vi "Server send.vi"() -> ()   [LabVIEW 2016, in "TCP文件传输系统.lvlib"]
uses:
  <vilib>/Utility/miscctls.llb/LVPointTypeDef.ctl
  <vilib>/Utility/sysdir.llb/System Directory Type.ctl
  <vilib>/Averna/Notify Icon/NotifyIcon.llb/BalloonIcon.ctl
  <vilib>/Averna/Notify Icon/NotifyIcon.llb/GetSelectedItemEvent.vi
  <vilib>/Averna/Notify Icon/NotifyIcon.llb/SetVisible.vi
  <vilib>/Averna/Notify Icon/NotifyIcon.llb/SetMenuDefaultItem.vi
  <vilib>/Averna/Notify Icon/NotifyIcon.llb/SetTipText.vi
  <vilib>/Averna/Notify Icon/NotifyIcon.llb/NotifyIcon.lvclass
panel:
  in  "选项卡控件":T1(tab)
  out "TCP发送全局簇":T2
  out "文件传输的路径":path
  in  "Application":string="版本升级文档.txt"
  in  "远程端口或服务名称":u16=11235
  out "本机网络地址":string="192.168.1.250"
  out "TCP发送全局簇 2":T2
  out "文件传输的路径 2":path
  in  "Application 2":string="update.exe"
  in  "远程端口或服务名称 2":u16=11236
  out "本机网络地址 2":string="192.168.1.250"
  out "TCP发送全局簇 3":T2
  out "文件传输的路径 3":path
  in  "Application 3":string="平台数据传输系统.exe"
  in  "远程端口或服务名称 3":u16=11234
  out "本机网络地址 3":string="192.168.1.250"
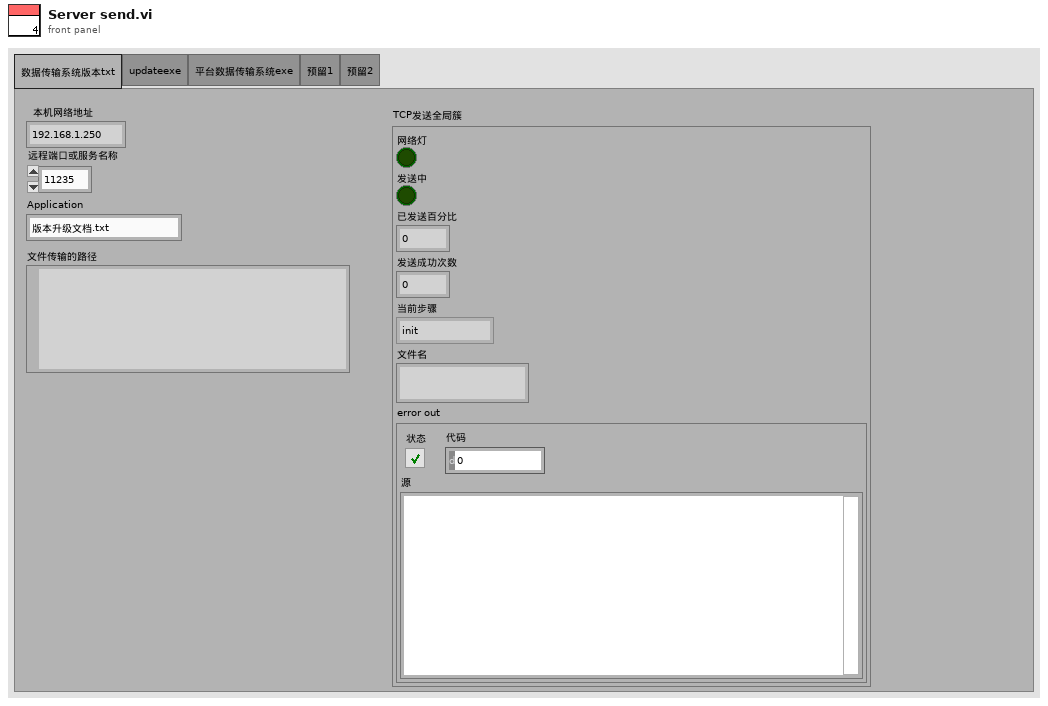
[diagram p1: front panel]
types:
  T1 = enum32{"数据传输系统版本txt", "updateexe", "平台数据传输系统exe", "预留1", "预留2"}
  T2 = cluster{"网络灯":bool, "发送中":bool, "已发送百分比":u8, "发送成功次数":dbl, "当前步骤":enum16{"init", "sendhead", "sendcontent", "sendsuccess", "over"}, "文件名":string, "error out":errorcluster}
  T3 = enum32{"Invalid", "Standard", "Closed", "Hidden", "Minimized", "Maximized"}
  T4 = typedef "LVPointTypeDef.ctl" = cluster{"Horizontal":i16, "Vertical":i16}
  T5 = typedef "NotifyIcon.lvlib/NotifyIcon.lvclass/BalloonIcon.ctl" = enum32{"None", "Information", "Warning", "Error"}
  T6 = typedef "System Directory Type.ctl" = i32
  T7 = enum32{"invalid app kind", "Development System", "Run Time System", "Student Edition", "Embedded LabVIEW", "Evaluation", "Custom"}
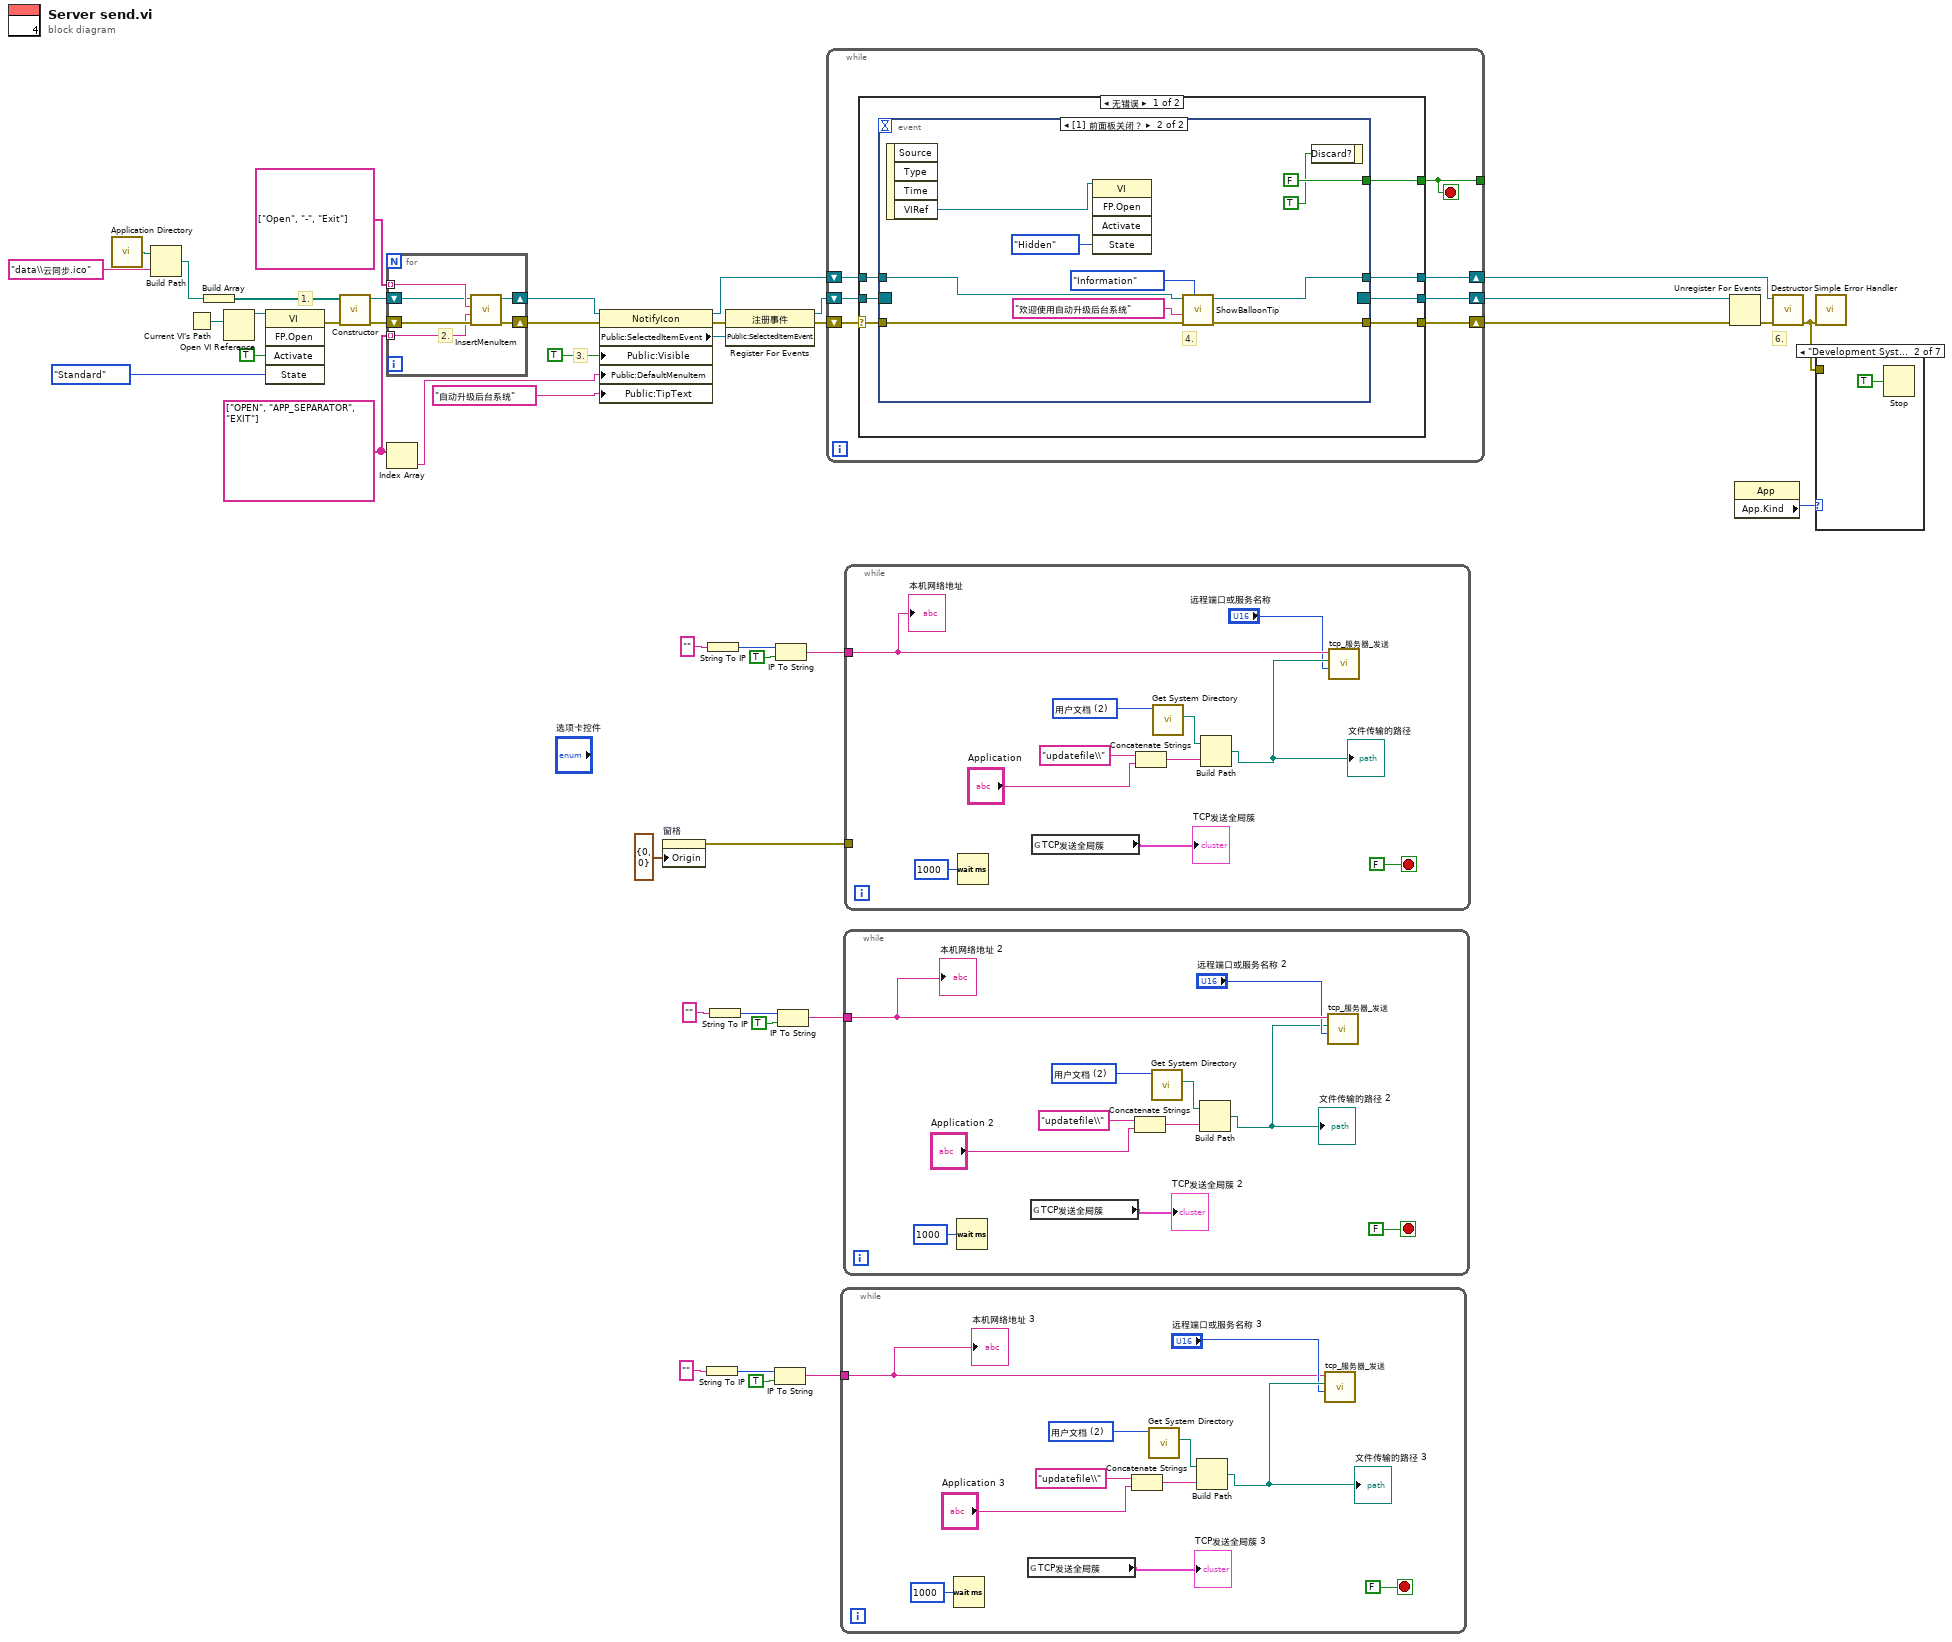
[diagram p0: block diagram]
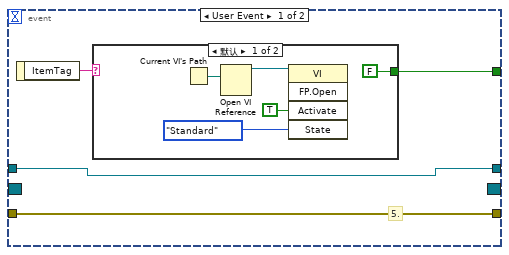
[diagram p2: hidden frame]
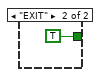
[diagram p3: hidden frame]
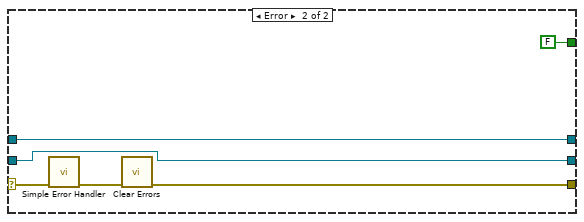
[diagram p4: hidden frame]
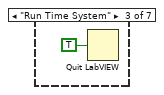
[diagram p6: hidden frame]
diagram:
  w13 = string[] ["OPEN", "APP_SEPARATOR", "EXIT"]
  # "6."
  # "3."
  # "1."
  n1 = call <vilib>:"Application Directory.vi"() -> ("Application Directory"=w11:path)
  n2 = Build Path(base path=w11, name or relative path="data\\云同步.ico" ("名称或相对路径")) -> (appended path=w21:path)
  n3 = Current VI's Path() -> (path=w8:path)
  n4 = Build Array(w21) -> (w16:path[])
  n5 = Open VI Reference(vi path=w8) -> (vi reference=w7:refnum<vi>)  [unwired: 5 in, 1 out]
  n6 = invoke class="VI" method="FP.Open"(reference=w7, "Activate"=TRUE ("激活？"), "State"=T3."Standard" ("状态")) -> (error out=w6:errorcluster)  [unwired: 2 in, 4 out]
  n7 = call <vilib>:"Constructor.vi"("error in"=w6, "IconFilePathList"=w16) -> ("error out"=w20:errorcluster, "NotifyIcon"=w12:refnum<class "NotifyIcon.lvclass">)  [unwired: 8 in]
  n8 = for {
    shift-right: [w48] -> w31
    shift-left: w20 -> [w49]
    tunnel: string[] ["Open", "-", "Exit"] -> [w47] mode=indexing
    tunnel: w13 -> [w46] mode=indexing
    shift-right: [w44] -> w30
    shift-left: w12 -> [w45]
    # "2."
    n9 = call <vilib>:"InsertMenuItem.vi"("error in"=w49, "ItemTag"=w46, "ItemName"=w47, "NotifyIcon in"=w45) -> ("error out"=w48:errorcluster, "NotifyIcon out"=w44:refnum<class "NotifyIcon.lvclass">)  [unwired: 6 in]
  }
  n10 = Index Array(array=w13) -> (element=w14:string)  [unwired: 1 in]
  n11 = property class="NotifyIcon"(reference=w30, error in=w31, "Public:Visible"=TRUE ("Visible"), "Public:DefaultMenuItem"=w14, "Public:TipText"="自动升级后台系统" ("TipText")) -> (reference out=w27:refnum<class "NotifyIcon.lvclass">, error out=w19:errorcluster, "Public:SelectedItemEvent"=w18:refnum<user-event>)
  n12 = property on="窗格" class="Pane"("Origin"=T4 {"Horizontal"=0, "Vertical"=0} ("原点")) -> (error out=w1:errorcluster)  [unwired: 2 in, 1 out]
  n13 = String To IP(1:"" ("名称")) -> (0:w34:u32)
  n14 = String To IP(1:"" ("名称")) -> (0:w41:u32)
  n15 = String To IP(1:"" ("名称")) -> (0:w37:u32)
  n16 = register-events(error in=w19, w18) -> (reference out=w3:refnum<event-registration>, error out=w4:errorcluster)  [unwired: 1 in]
  n17 = IP To String(1:TRUE ("句点符号？(F)"), 2:w34) -> (0:w35:string)
  n18 = IP To String(1:TRUE ("句点符号？(F)"), 2:w41) -> (0:w40:string)
  n19 = IP To String(1:TRUE ("句点符号？(F)"), 2:w37) -> (0:w36:string)
  n20 = while {
    shift-right: [w53] -> w25
    shift-left: w4 -> [w52]
    shift-right: [w54] -> w23
    shift-left: w27 -> [w55]
    shift-right: [w51] -> w24
    shift-left: w3 -> [w56]
    tunnel: [w50] -> _
    stop <- w50 stop-if-true
    n21 = case shown="无错误" w52 {
      selector: w52 -> [w58 w89]
      tunnel: w56 -> [w63 w84]
      tunnel: w55 -> [w62 w85]
      tunnel: [w61 w85] -> w54
      tunnel: [w60 w87] -> w53
      tunnel: [w59 FALSE ("Discard?")] -> w50
      tunnel: [w57 w84] -> w51
      frame No Error {
        n22 = event shown="[1] 前面板关闭？" {
          selector: w63 -> [_ _]
          dyn-events: [_ _] -> w57
          timeout: _ -> [_ _]
          tunnel: w58 -> [w66 w82]
          tunnel: [w66 w81] -> w60
          tunnel: [w65 FALSE ("Discard?")] -> w59
          tunnel: w62 -> [w64 w83]
          tunnel: [w64 w80] -> w61
          event User Event {
            # "5."
            n23 = event-data() -> ("ItemTag"=w67:string)  [unwired: 1 in]
            n24 = case shown="默认" w67 {
              tunnel: [FALSE TRUE] -> w65
              frame Default {
                n25 = Current VI's Path() -> (path=w69:path)
                n26 = Open VI Reference(vi path=w69) -> (vi reference=w70:refnum<vi>)  [unwired: 5 in, 1 out]
                n27 = invoke class="VI" method="FP.Open"(reference=w70, "Activate"=TRUE ("激活？"), "State"=T3."Standard" ("状态")) -> ()  [unwired: 2 in, 5 out]
              }
              frame "EXIT" {
              }
            }
          }
          event Panel Close? {
            # "4."
            n28 = event-data() -> ("VIRef"=w76:refnum<vi>)  [unwired: 1 in, 3 out]
            n29 = invoke class="VI" method="FP.Open"(reference=w76, "State"=T3."Hidden" ("状态")) -> ()  [unwired: 3 in, 5 out]
            n30 = call <vilib>:"ShowBalloonTip.vi"("Balloon Icon"=BalloonIcon."Information", "error in"=w82, "Text"="欢迎使用自动升级后台系统", "NotifyIcon in"=w83) -> ("error out"=w81:errorcluster, "NotifyIcon out"=w80:refnum<class "NotifyIcon.lvclass">)  [unwired: 6 in]
            n31 = event-data("Discard?"=TRUE ("放弃？")) -> ()  [unwired: 1 in, 1 out]
          }
        }
      }
      frame Error {
        n32 = call <vilib>:"Simple Error Handler.vi"("error in (no error)"=w89) -> ("error out"=w88:errorcluster)  [unwired: 4 in, 4 out]
        n33 = call <vilib>:"Clear Errors.vi"("error in (no error)"=w88) -> ("error out"=w87:errorcluster)  [unwired: 5 in, 1 out]
      }
    }
  }
  n34 = while {
    tunnel: w35 -> [w92]
    stop <- FALSE stop-if-true
    w99 = T6 2 items=["用户目录"=0, "用户桌面"=1, "用户文档"=2, "用户应用程序数据"=3, "用户设置"=4, "用户临时目录"=5, "公共文档"=6, "公共应用程序数据"=7, "公共设置"=8, "公共缓存"=13, "系统核心库"=9, "系统安装库"=10, "应用程序文件"=11, "启动盘根目录"=12] ("system directory type")
    n35 = Wait (ms)(milliseconds to wait=u32 1000 ("等待时间（毫秒）")) -> ()  [unwired: 1 out]
    n36 = global read "全局变量1.vi" "TCP发送全局簇"() -> (→"TCP发送全局簇 3":T2)
    n37 = Concatenate Strings("updatefile\\" ("condition"), "Application 3") -> (w98:string)
    n38 = call <vilib>:"Get System Directory.vi"("system directory type"=w99) -> ("system directory"=w96:path)  [unwired: 10 in]
    n39 = Build Path(base path=w96, name or relative path=w98) -> (appended path=w94:path)
    "文件传输的路径 3" <- w94
    n40 = call "tcp_服务器_发送.vi"("远程端口或服务名称"="远程端口或服务名称 3", "原文件路径（使用对话框）"=w94, "服务器网络地址"=w92) -> ()  [unwired: 9 in]
    "本机网络地址 3" <- w92
  }
  n41 = while {
    tunnel: w36 -> [w105]
    stop <- FALSE stop-if-true
    w110 = T6 2 items=["用户目录"=0, "用户桌面"=1, "用户文档"=2, "用户应用程序数据"=3, "用户设置"=4, "用户临时目录"=5, "公共文档"=6, "公共应用程序数据"=7, "公共设置"=8, "公共缓存"=13, "系统核心库"=9, "系统安装库"=10, "应用程序文件"=11, "启动盘根目录"=12] ("system directory type")
    n42 = Wait (ms)(milliseconds to wait=u32 1000 ("等待时间（毫秒）")) -> ()  [unwired: 1 out]
    n43 = global read "全局变量1.vi" "TCP发送全局簇"() -> (→"TCP发送全局簇 2":T2)
    n44 = Concatenate Strings("updatefile\\" ("condition"), "Application 2") -> (w109:string)
    n45 = call <vilib>:"Get System Directory.vi"("system directory type"=w110) -> ("system directory"=w107:path)  [unwired: 10 in]
    n46 = Build Path(base path=w107, name or relative path=w109) -> (appended path=w101:path)
    "文件传输的路径 2" <- w101
    n47 = call "tcp_服务器_发送.vi"("远程端口或服务名称"="远程端口或服务名称 2", "原文件路径（使用对话框）"=w101, "服务器网络地址"=w105) -> ()  [unwired: 9 in]
    "本机网络地址 2" <- w105
  }
  n48 = while {
    tunnel: w40 -> [w120]
    tunnel: w1 -> [_]
    stop <- FALSE stop-if-true
    w121 = T6 2 items=["用户目录"=0, "用户桌面"=1, "用户文档"=2, "用户应用程序数据"=3, "用户设置"=4, "用户临时目录"=5, "公共文档"=6, "公共应用程序数据"=7, "公共设置"=8, "公共缓存"=13, "系统核心库"=9, "系统安装库"=10, "应用程序文件"=11, "启动盘根目录"=12] ("system directory type")
    n49 = Wait (ms)(milliseconds to wait=u32 1000 ("等待时间（毫秒）")) -> ()  [unwired: 1 out]
    n50 = global read "全局变量1.vi" "TCP发送全局簇"() -> (→"TCP发送全局簇":T2)
    n51 = Concatenate Strings("updatefile\\" ("condition"), "Application") -> (w119:string)
    n52 = call <vilib>:"Get System Directory.vi"("system directory type"=w121) -> ("system directory"=w117:path)  [unwired: 10 in]
    n53 = Build Path(base path=w117, name or relative path=w119) -> (appended path=w116:path)
    "文件传输的路径" <- w116
    n54 = call "tcp_服务器_发送.vi"("远程端口或服务名称"="远程端口或服务名称", "原文件路径（使用对话框）"=w116, "服务器网络地址"=w120) -> ()  [unwired: 9 in]
    "本机网络地址" <- w120
  }
  n55 = Unregister For Events(event registration refnum=w24, error in=w25) -> (error out=w26:errorcluster)
  n56 = property class="App"() -> ("App.Kind"=w5:T7)  [unwired: 2 in, 2 out]
  n57 = call <vilib>:"Destructor.vi"("error in"=w26, "NotifyIcon"=w23) -> ("error out"=w22:errorcluster)  [unwired: 9 in]
  n58 = call <vilib>:"Simple Error Handler.vi"("error in (no error)"=w22) -> ()  [unwired: 4 in, 5 out]
  n59 = case shown="\"Development System\"" w5 {
    tunnel: w22 -> [_ _ _ _ _ _ _]
    frame "invalid app kind", Default {
    }
    frame "Development System" {
      n60 = Stop(stop? (T)=TRUE ("可见")) -> ()
    }
    frame "Run Time System" {
      n61 = Quit LabVIEW(quit? (T)=TRUE ("退出？(T)")) -> ()
    }
    frame "Student Edition" {
    }
    frame "Embedded LabVIEW" {
    }
    frame "Evaluation" {
    }
    frame "Custom" {
    }
  }
